vi "main_poly.vi"() -> ()   [LabVIEW 2011]
uses:
  floatToString.vi
  booleanToString.vi
panel:
  in  "Label.Size:Height":u32(knob) scale=0.0..100.0
  in  "Label.Colors:BG Color":u32(slide) scale=0.0..16000000.0
  out "Knob":dbl
  out "data":bool
  out "Numeric":dbl
  out "ClassName":string[](array[string])
  out "Data String":string[](array[string])
  out "type string":i16[][](array[numeric])
  out "Ctl Refnum":refnum<vi>
  out "Knob":string
  out "OK Button":string
  in  "srcCluster":T1 {"Knob" scale=0.0..10.0}
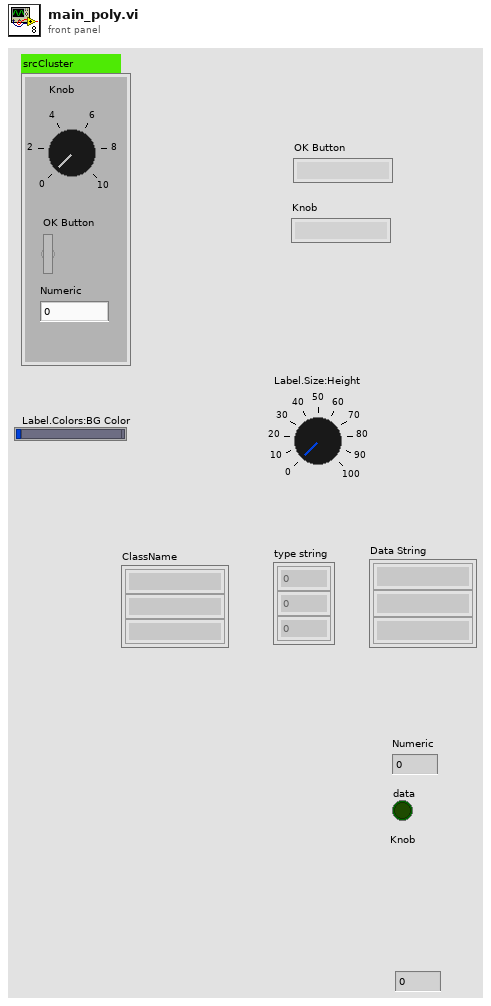
[diagram p1: front panel]
types:
  T1 = cluster{"OK Button":bool, "Knob":dbl, "Numeric":dbl}
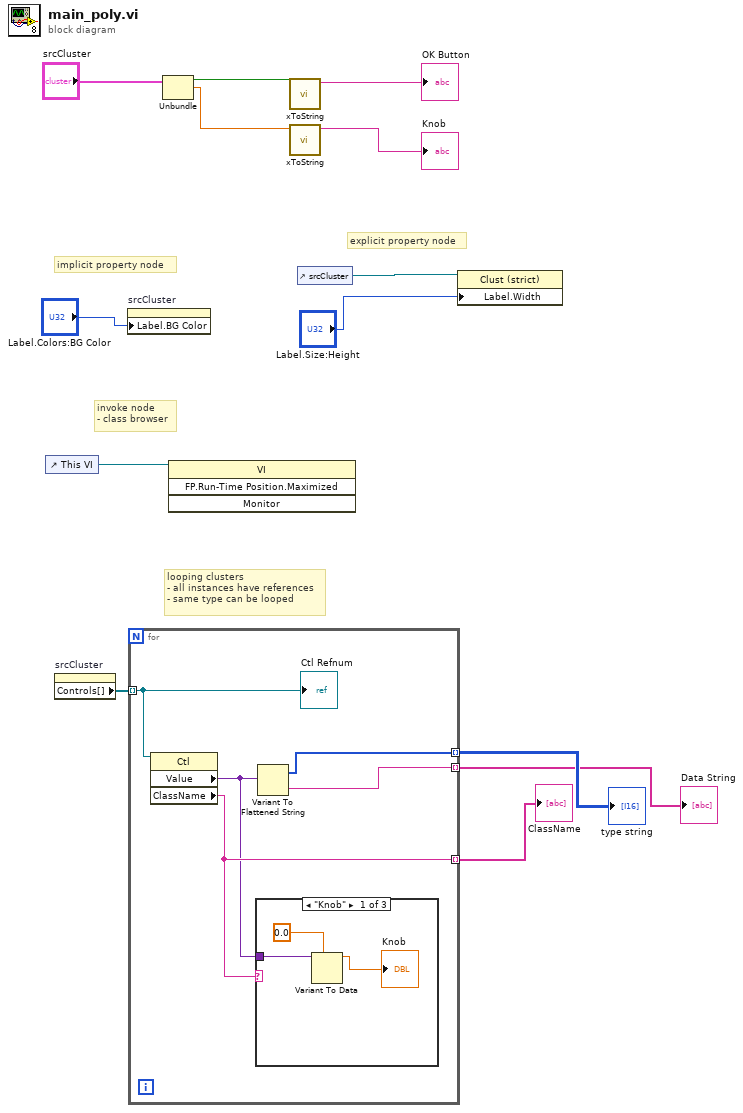
[diagram p0: block diagram]
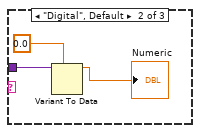
[diagram p2: hidden frame]
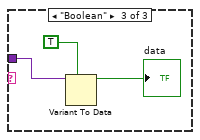
[diagram p3: hidden frame]
diagram:
  # "looping clusters\n- all instances have references\n- same type can be looped"
  # "invoke node\n- class browser"
  # "explicit property node"
  # "implicit property node"
  n1 = control-ref of="This VI"() -> (w3:refnum<vi>)
  n2 = property on="srcCluster" class="Clust (strict)"() -> ("Controls[]"=w8:refnum<vi>[])  [unwired: 2 in, 2 out]
  n3 = property on="srcCluster" class="Clust (strict)"("Label.BG Color"="Label.Colors:BG Color") -> ()  [unwired: 2 in, 2 out]
  n4 = for {
    tunnel: w8 -> [w18] mode=indexing
    tunnel: [w17] -> w7 mode=indexing
    tunnel: [w16] -> w6 mode=indexing
    tunnel: [w15] -> w5 mode=indexing
    n5 = property class="Ctl"(reference=w18) -> ("Value"=w14:variant, "ClassName"=w15:string)  [unwired: 1 in, 2 out]
    n6 = case shown="\"Knob\"" w15 {
      tunnel: w14 -> [w19 w24 w26]
      frame "Knob" {
        n7 = Variant To Data(type=0.0, Variant=w19) -> (data=→"Knob":dbl)  [unwired: 1 in, 1 out]
      }
      frame "Digital", Default {
        n8 = Variant To Data(type=0.0, Variant=w24) -> (data=→"Numeric":dbl)  [unwired: 1 in, 1 out]
      }
      frame "Boolean" {
        n9 = Variant To Data(type=TRUE, Variant=w26) -> (data=→"data":bool)  [unwired: 1 in, 1 out]
      }
    }
    n10 = Variant To Flattened String(Variant=w14) -> (data string=w16:string, 1:w17:i16[])
    "Ctl Refnum" <- w18
  }
  "type string" <- w7
  "Data String" <- w6
  "ClassName" <- w5
  n11 = Unbundle("srcCluster") -> ("OK Button"=w13:bool, "Knob"=w11:dbl)  [unwired: 1 out]
  n12 = invoke class="VI" method="FP.Run-Time Position.Maximized"(reference=w3) -> ()  [unwired: 3 in, 4 out]
  n13 = call-poly "xToString.vi"("Boolean"=w13) -> ("String"=→"OK Button":string)  [unwired: 10 in]
  n14 = call-poly "xToString.vi"("Numeric"=w11) -> ("String"=→"Knob":string)  [unwired: 10 in]
  n15 = control-ref of="srcCluster"() -> (w2:refnum<vi>)
  n16 = property class="Clust (strict)"(reference=w2, "Label.Width"="Label.Size:Height") -> ()  [unwired: 1 in, 2 out]
